vi "Write VI name.vi"(8 "error in":errorcluster, 10 "VI name":string, 11 "io configuration in":refnum<class "io configuration.lvclass">) -> (0 "error out":errorcluster, 3 "io configuration out":refnum<class "io configuration.lvclass">)   [LabVIEW 2015, in "io configuration.lvclass"]
uses:
  io configuration.lvclass
  io configuration.lvclass/io configuration.ctl
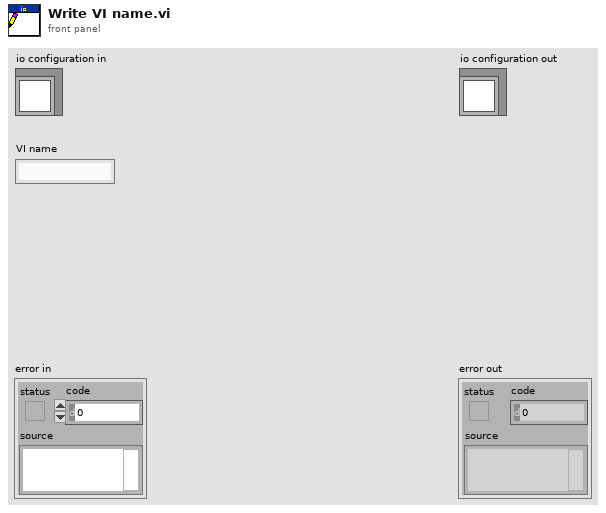
[diagram p1: front panel]
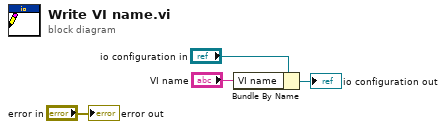
[diagram p0: block diagram]
diagram:
  n1 = Bundle By Name(cluster="io configuration in", "VI name"="VI name") -> (→"io configuration out":refnum<class "io configuration.lvclass">)
  "error out" <- "error in"
